vi "Launch GPS Actor.vi"(7 "Sim?":bool, 11 "RDS Root Actor in":refnum<class "RDS Root Actor.lvclass">) -> (3 "RDS Root Actor out":refnum<class "RDS Root Actor.lvclass">)   [LabVIEW 2015, in "RDS Root Actor.lvlib" / "RDS Root Actor.lvclass"]
uses:
  RDS Root Actor.lvclass
  GPS Instrument/GPS Instrument/GPS Instrument.lvclass
  Libraries/RDS Framework/RDS Message ID.ctl
  Libraries/RDS Instruments/RDS Instrument Enums.ctl
  RDS Parent Actor/RDS Parent Actor/RDS Parent Actor.lvclass/RDS Parent Actor.ctl
  RDS Serial Instrument Actor/RDS Serial Instrument Actor.lvclass/RDS Serial Instrument Actor.ctl
  Sim GPS/Sim GPS/Sim GPS.lvclass
  RDS Parent Actor/RDS Parent Actor/RDS Parent Actor.lvclass
  RDS Serial Instrument Actor/RDS Serial Instrument Actor.lvclass
  Libraries/RDS Child Messages/RDS Child Messages.lvlib
  Libraries/Configuration Library/RDS Configuration Library.lvlib
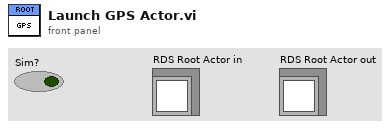
[diagram p1: front panel]
types:
  T1 = typedef "RDS Configuration Library.lvlib/RDS Instrument Enums.ctl" = enum16{"AIP", "GPS", "Compass", "PORT Motor", "STBD Motor", "LSR", "Depth Transducer", "BTB"}
  T2 = typedef "RDS Child Messages.lvlib/RDS Message ID.ctl" = enum16{"RDS Hello World", "String Message", "AIP_Status", "AIP_Command", "GPS_Data", "MCB_Command", "MCB_Status", "Compass_Data", "Depth_Data", "Battery_Data", "Contoller_State", "Set_Mag_Dev", "BTB_Shutdown", "State_Sample_Request", "State_Sample", "PID_Gains_Set", "Helm_Limiter_Set", "Helm_Heading_Command", "Helm_Steering_Command", "Helm_Status", "Controller_Message", "AIP_Set_Min_Depth", "Mission_Controller_State", "Mission_Upload", "Mission_Set_Op_and_Run", "Mission_Settings_Set"}
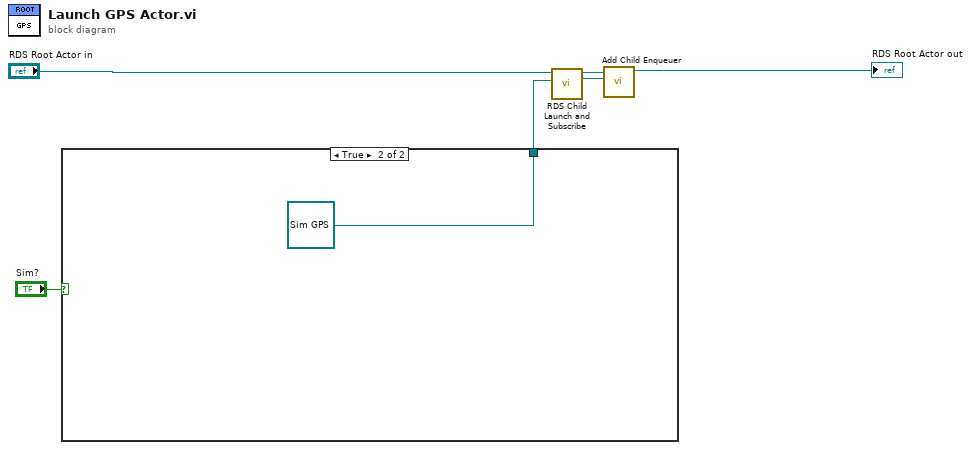
[diagram p0: block diagram]
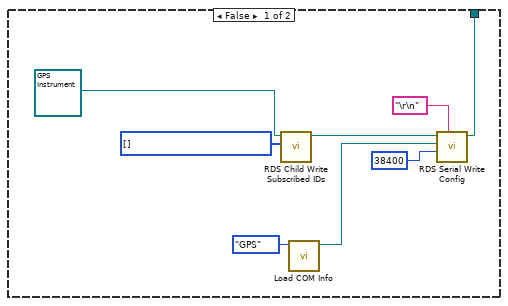
[diagram p2: hidden frame]
diagram:
  n1 = case shown="True" "Sim?" {
    tunnel: [w14 refnum<class "Sim GPS.lvclass"> refnum ("Sim GPS.lvlib:Sim GPS.lvclass")] -> w2
    frame False {
      w9 = T2[] [] items=["RDS Hello World", "String Message", "AIP_Status", "AIP_Command", "GPS_Data", "MCB_Command", "MCB_Status", "Compass_Data", "Depth_Data", "Battery_Data", "Contoller_State", "Set_Mag_Dev", "BTB_Shutdown", "State_Sample_Request", "State_Sample", "PID_Gains_Set", "Helm_Limiter_Set", "Helm_Heading_Command", "Helm_Steering_Command", "Helm_Status", "Controller_Message", "AIP_Set_Min_Depth", "Mission_Controller_State", "Mission_Upload", "Mission_Set_Op_and_Run", "Mission_Settings_Set"] ("Subscribed IDs")
      n2 = call "RDS Child Write Subscribed IDs.vi"("Subscribed IDs"=w9, "RDS Parent Actor in"=refnum<class "GPS Instrument.lvclass"> refnum ("GPS Instrument.lvlib:GPS Instrument.lvclass")) -> ("RDS Parent Actor out"=w11:refnum<class "GPS Instrument.lvclass">)  [unwired: 8 in, 1 out]
      n3 = call "Load COM Info.vi"("Serial Instrument"=RDS_Instrument_Enums."GPS") -> ("COM Port"=w7:refnum<visa-resource-name>)  [unwired: 10 in]
      n4 = call "RDS Serial Write Config.vi"("Termination Char(s)"="\r\n", "baud rate"=u32 38400, "VISA resource name"=w7, "RDS Serial Instrument Actor in"=w11) -> ("RDS Serial Instrument Actor out"=w14:refnum<class "GPS Instrument.lvclass">)  [unwired: 6 in, 1 out]
    }
    frame True {
    }
  }
  n5 = call "RDS Child Launch and Subscribe.vi"("RDS Child in"=w2, "Caller Actor in"="RDS Root Actor in") -> ("Nested Actor's Enqueuer"=w5:refnum<class "Message Enqueuer.lvclass">, "Caller Actor Out"=w4:refnum<class "RDS Root Actor.lvclass">)  [unwired: 7 in, 1 out]
  n6 = call "Add Child Enqueuer.vi"("Nested Actor's Enqueuer"=w5, "RDS Root Actor in"=w4) -> ("RDS Root Actor out"=→"RDS Root Actor out":refnum<class "RDS Root Actor.lvclass">)  [unwired: 8 in, 1 out]
